vi "CovarianceofPointSetsA&B.vi"(8 "error in (no error)":errorcluster, 9 "A - mean(A)":dbl[][](array[numeric]), 11 "B - mean(B)":dbl[][](array[numeric])) -> (0 "error out":errorcluster, 3 "Covariance":T1)   [LabVIEW 2020, in "pointset_utils.lvlib" / "Affine Estimation.lvlib"]
uses:
  Affine Estimation.lvlib
  <vilib>/Analysis/Matrix/Datatypes/RealMatrix.ctl
  <vilib>/Analysis/baseanly.llb/Real A x B.vi
  <vilib>/Analysis/Matrix/NI_Matrix.lvlib
  <vilib>/Analysis/NI_AALBase.lvlib
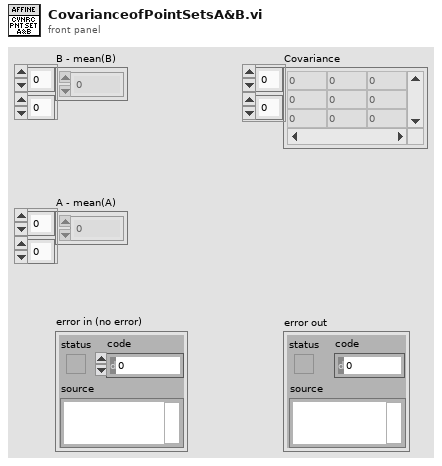
[diagram p1: front panel]
types:
  T1 = typedef "NI_Matrix.lvlib/RealMatrix.ctl" = dbl[][]
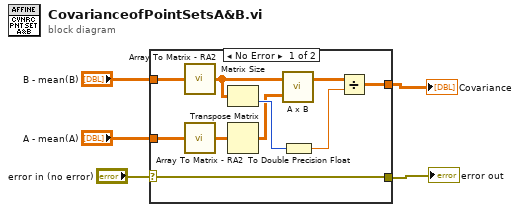
[diagram p0: block diagram]
diagram:
  n1 = case shown="No Error" "error in (no error)" {
    selector: "error in (no error)" -> [w6 w16]
    tunnel: "A - mean(A)" -> [w15 _]
    tunnel: [w14 _] -> w4
    tunnel: "B - mean(B)" -> [w11 _]
    tunnel: [w6 w16] -> w1
    frame No Error {
      n2 = call <vilib>:"Array To Matrix - RA2.vi"("Real 2D Array"=w11) -> ("Real Matrix"=w12:T1)
      n3 = call <vilib>:"Array To Matrix - RA2.vi"("Real 2D Array"=w15) -> ("Real Matrix"=w7:T1)
      n4 = Matrix Size(0:w12) -> (2:w13:i32)  [unwired: 1 out]
      n5 = Transpose Matrix(1:w7) -> (0:w8:T1)
      n6 = call-poly <vilib>:"A x B.vi"("B"=w8, "A"=w12) -> ("A x B"=w9:T1)  [unwired: 1 out]
      n7 = To Double Precision Float(number=w13) -> (double precision float=w10:dbl)
      n8 = Divide(x=w9, y=w10) -> (x/y=w14:T1)
    }
    frame Error {
    }
  }
  "Covariance" <- w4
  "error out" <- w1
